vi "num2String.vi"(1 "Precision (1-6)":i16, 2 "Number":dbl format="%#_13g") -> (0 "F-format String":string)   [LabVIEW 2013]
panel:
  # "Notes:\n1. Ideally include this VI with sample2String\n2. Build on this VI to include various number to string conversions"
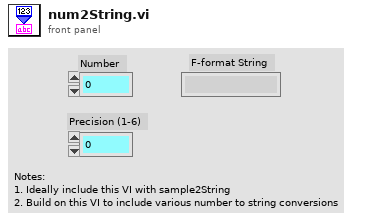
[diagram p1: front panel]
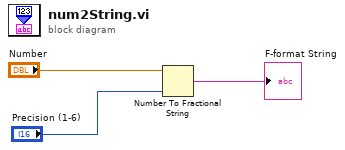
[diagram p0: block diagram]
diagram:
  n1 = Number To Fractional String(number="Number", precision (6)="Precision (1-6)") -> (F-format string=→"F-format String":string)  [unwired: 2 in]
